vi "SWI Panel.vi"(8 "error in (no error)":errorcluster, 9 "SWI Configuration (\"\")":string, 10 "SWI Position In":variant, 11 "SWI Command":T1) -> (0 "error out":errorcluster, 1 "SWI Flat Output":string, 2 "SWI Position Out":variant)   [LabVIEW 2011]
uses:
  SWI Command.ctl
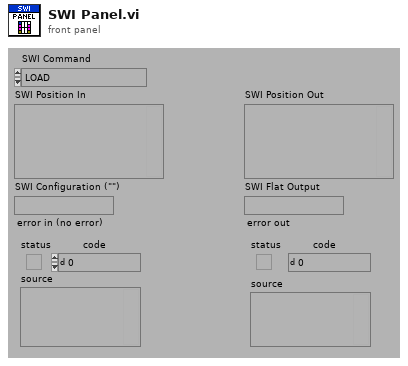
[diagram p1: front panel]
types:
  T1 = typedef "SWI Command.ctl" = enum16{"LOAD", "INITIALIZE", "PRESET", "SET STIMULUS", "GET STIMULUS", "GET INFO", "RELEASE", "UNLOAD"}
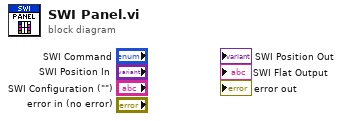
[diagram p0: block diagram]
diagram:
